vi "Pixel_Trigger_Main.vi"(8 "Counter(s)":tag="Dev1/ctr0", 9 "Number Of Pulses":i32=5, 10 "Frequency":dbl=10000.0, 11 "Source":tag="/Dev1/PFI9" caption="Trigger Source") -> (0 "error out":errorcluster, 3 "task out":refnum<k21>)   [LabVIEW 2009]
uses:
  <vilib>/DAQmx/configure/trigger.llb/DAQmx Start Trigger (Digital Edge).vi
  <vilib>/DAQmx/configure/timing.llb/DAQmx Timing (Implicit).vi
  <vilib>/DAQmx/create/channels.llb/DAQmx Create Channel (CO-Pulse Generation-Frequency).vi
  Program Files/National Instruments/LabVIEW 2009/resource/objmgr/daqmx.rc
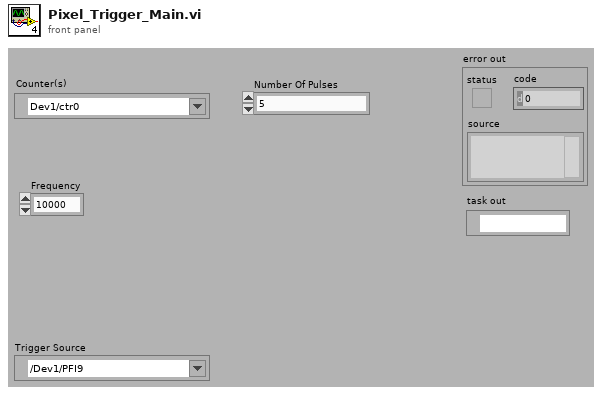
[diagram p1: front panel]
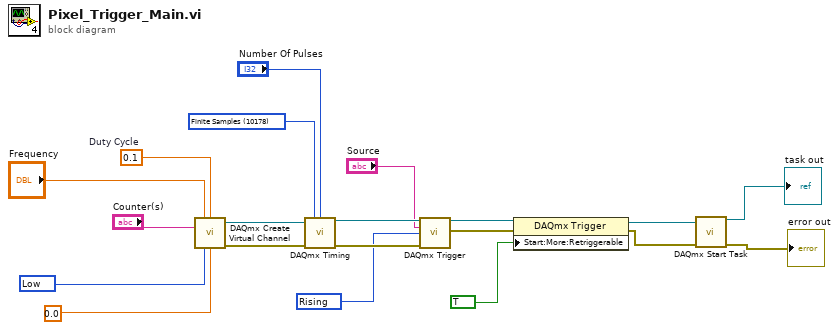
[diagram p0: block diagram]
diagram:
  w9 = 10280 items=["Rising"=10280, "Falling"=10171] ("Trigger Edge")
  w16 = 10214 items=["High"=10192, "Low"=10214] ("Idle State")
  w13 = 0.1  # Duty Cycle
  w18 = 10178 items=["Finite Samples"=10178, "Continuous Samples"=10123] ("sample mode")
  n1 = call-poly <vilib>:"DAQmx Create Virtual Channel.vi"("frequency"="Frequency", "duty cycle"=w13, "counter"="Counter(s)", "idle state"=w16, "initial delay"=0.0 ("Initial delay")) -> ("task out"=w19:refnum<k21>, "error out"=w20:errorcluster)  [unwired: 4 in, 5 out]
  n2 = call-poly <vilib>:"DAQmx Timing.vi"("task/channels in"=w19, "sample mode"=w18, "samples per channel"="Number Of Pulses", "error in"=w20) -> ("task out"=w12:refnum<k21>, "error out"=w11:errorcluster)  [unwired: 2 in, 8 out]
  n3 = call-poly <vilib>:"DAQmx Trigger.vi"("task/channels in"=w12, "source"="Source", "edge"=w9, "error in"=w11) -> ("task out"=w7:refnum<k21>, "error out"=w6:errorcluster)  [unwired: 10 out]
  n4 = property class="DAQmx Trigger"(reference=w7, error in=w6, "Start:More:Retriggerable"=TRUE) -> (reference out=w2:refnum<k21>, error out=w5:errorcluster)
  n5 = call <vilib>:"DAQmx Start Task.vi"("task/channels in"=w2, "error in"=w5) -> ("task out"=→"task out":refnum<k21>, "error out"=→"error out":errorcluster)  [unwired: 12 out]
